vi "getBalanceGyro.vi"() -> (3 "BalanceGyroReading":dbl)   [LabVIEW 2020]
uses:
  DriveGlobals.vi
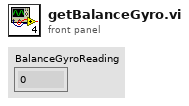
[diagram p1: front panel]
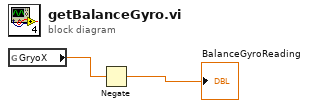
[diagram p0: block diagram]
diagram:
  n1 = global read "DriveGlobals.vi" "GryoX"() -> (w2:dbl)
  n2 = Negate(x=w2) -> (-x=→"BalanceGyroReading":dbl)
